vi "Init.vi"(8 "error in (no error)":errorcluster, 11 "Modbus TCP Micro Master in":refnum<class "Modbus TCP Micro Master.lvclass">) -> (0 "error out":errorcluster, 3 "Modbus TCP Micro Master out":refnum<class "Modbus TCP Micro Master.lvclass">)   [LabVIEW 2023, in "Modbus TCP Micro.lvlib" / "Modbus TCP Micro Master.lvclass"]
uses:
  Modbus TCP Micro Master.lvclass
  Modbus TCP Micro Master.lvclass/Modbus TCP Micro Master.ctl
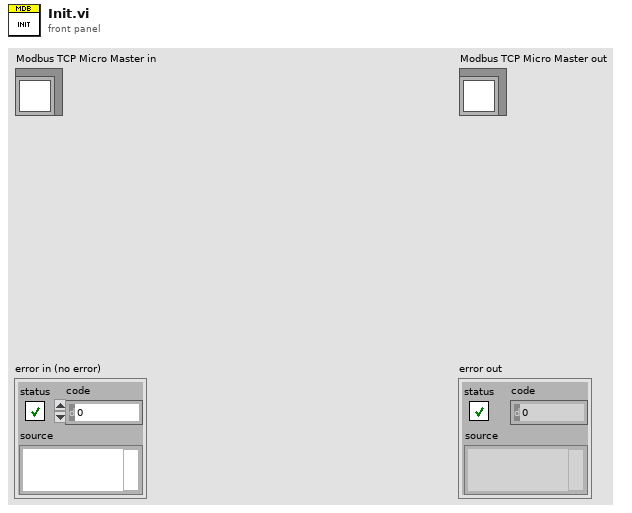
[diagram p1: front panel]
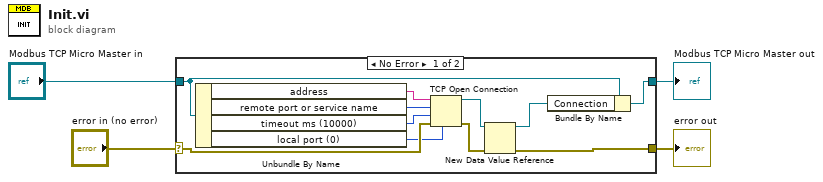
[diagram p0: block diagram]
diagram:
  n1 = case shown="No Error" "error in (no error)" {
    selector: "error in (no error)" -> [w15 w17]
    tunnel: [w7 w17] -> w3
    tunnel: [w14 w16] -> w1
    tunnel: "Modbus TCP Micro Master in" -> [w13 w16]
    frame No Error {
      n2 = Unbundle By Name(w13) -> ("address"=w12:string, "remote port or service name"=w11:u16, "timeout ms (10000)"=w10:i32, "local port (0)"=w9:u16)
      n3 = TCP Open Connection(address=w12, remote port or service name=w11, timeout ms (60000)=w10, local port=w9, error in (no error)=w15) -> (connection ID=w6:refnum<k5>, error out=w8:errorcluster)
      n4 = New Data Value Reference(data value=w6, error in=w8) -> (data value reference=w5:refnum<data-value>, error out=w7:errorcluster)
      n5 = Bundle By Name(cluster=w13, "Connection"=w5) -> (w14:refnum<class "Modbus TCP Micro Master.lvclass">)
    }
    frame Error {
    }
  }
  "error out" <- w3
  "Modbus TCP Micro Master out" <- w1
